vi "TDMSchannellist.vi"(11 "file path":path) -> (0 "channel list":string, 3 "channel aray":string[](array[string]), 7 "group":string)   [LabVIEW 2015]
panel:
  in  "data type":waveform(dbl)[](array[waveform])
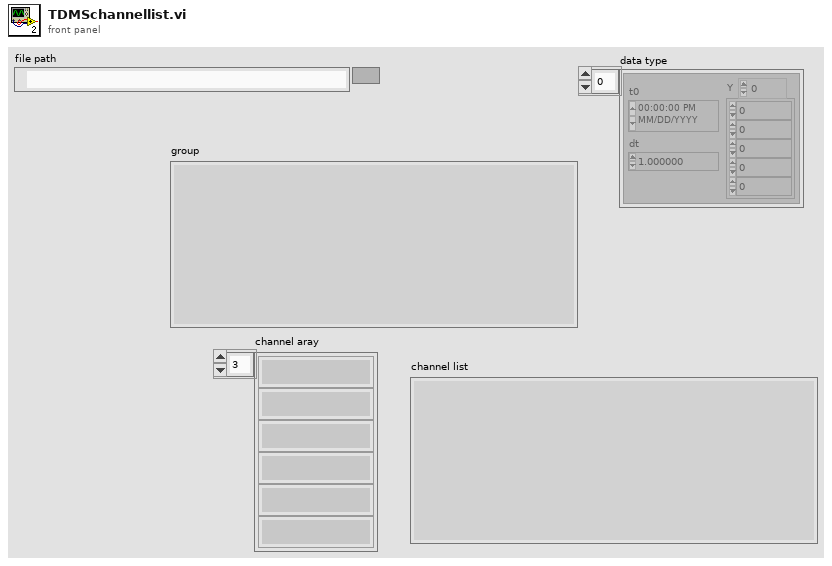
[diagram p1: front panel]
types:
  T1 = enum16{"open", "open or create", "create or replace", "create", "open (read-only)"}
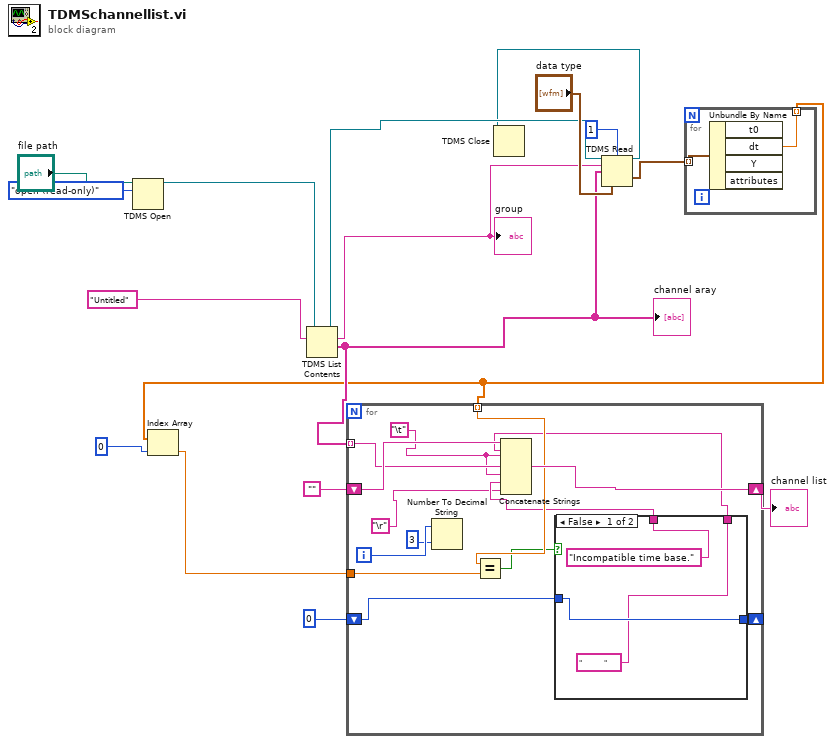
[diagram p0: block diagram]
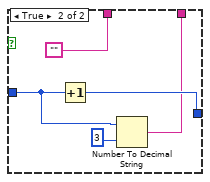
[diagram p2: hidden frame]
diagram:
  n1 = TDMS Open(10:T1."open (read-only)" ("operation (0:open)"), 11:"file path") -> (3:w16:refnum<k34>)  [unwired: 5 in, 1 out]
  n2 = TDMS List Contents(6:"Untitled" ("Group name"), 7:w16) -> (1:w9:string[], 2:w2:string, 3:w5:refnum<k34>)  [unwired: 1 in, 1 out]
  "group" <- w2
  "channel aray" <- w9
  n3 = TDMS Read(0:w5, 2:i64 1 ("count (-1: all)"), 5:w2, 7:w9, 12:"data type") -> (4:w4:refnum<k34>, 10:w10:waveform(dbl)[])  [unwired: 3 in, 4 out]
  n4 = TDMS Close(11:w4) -> ()  [unwired: 1 in, 2 out]
  n5 = for {
    tunnel: w10 -> [w19] mode=indexing
    tunnel: [w18] -> w7 mode=indexing
    n6 = Unbundle By Name(w19) -> ("dt"=w18:dbl)  [unwired: 3 out]
  }
  n7 = Index Array(array=w7, index=0) -> (element=w6:dbl)
  n8 = for {
    tunnel: w9 -> [w31] mode=indexing
    shift-right: [w32] -> w13
    shift-left: "" -> [w33]
    tunnel: w7 -> [w27] mode=indexing
    tunnel: w6 -> [w28]
    shift-right: [w21] -> _
    shift-left: 0 -> [w22]
    i -> [w30]
    w25 = "\t"
    n9 = Number To Decimal String(number=w30, width (-)=3) -> ()  [unwired: 1 out]
    n10 = Equal?(x=w27, y=w28) -> (x = y?=w26:bool)
    n11 = case shown="False" w26 {
      tunnel: ["Incompatible time base." ("Group name") ""] -> w24
      tunnel: w22 -> [w35 w38]
      tunnel: [w35 w40] -> w21
      tunnel: ["           " ("Group name") w37] -> w20
      frame False {
      }
      frame True {
        n12 = Increment(x=w38) -> (x+1=w40:i32)
        n13 = Number To Decimal String(number=w38, width (-)=3) -> (decimal integer string=w37:string)
      }
    }
    n14 = Concatenate Strings(w33, w20, w25, w31, w25, w24, "\r") -> (w32:string)
  }
  "channel list" <- w13
